vi "R&S RF Off.vi"() -> (0 "Error":bool)   [LabVIEW 2009]
doc: "This device configures the Rohde & Schwarz RF Generator for use. The central frequency, modulation, RF power, and GPIB address are taken from the QCA Global."
uses:
  QCA Global.vi
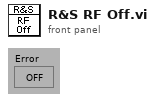
[diagram p1: front panel]
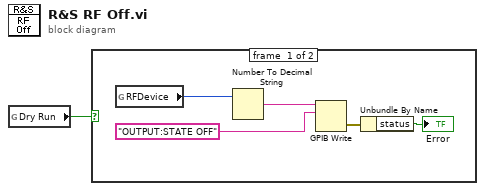
[diagram p0: block diagram]
diagram:
  n1 = global read "QCA Global.vi" "Dry Run"() -> (w1:bool)
  n2 = case shown="False" w1 {
    frame #0 {
      n3 = global read "QCA Global.vi" "RFDevice"() -> (w4:i32)
      n4 = Number To Decimal String(number=w4) -> (decimal integer string=w3:string)  [unwired: 1 in]
      n5 = GPIB Write(0:w3, 1:"OUTPUT:STATE OFF") -> (6:w6:errorcluster)  [unwired: 3 in, 1 out]
      n6 = Unbundle By Name(w6) -> ("status"=→"Error":bool)
    }
    frame #1 {
    }
  }
